vi "Get Attribute I32.vi"(8 "error in":errorcluster, 10 "Attribute":string, 11 "Config from Excel Table in":refnum<class "Config from Excel Table.lvclass">) -> (0 "error out":errorcluster, 2 "Value":i32, 3 "Config from Excel Table out":refnum<class "Config from Excel Table.lvclass">)   [LabVIEW 2025, in "Config from Excel Table.lvclass"]
uses:
  Config from Excel Table.lvclass
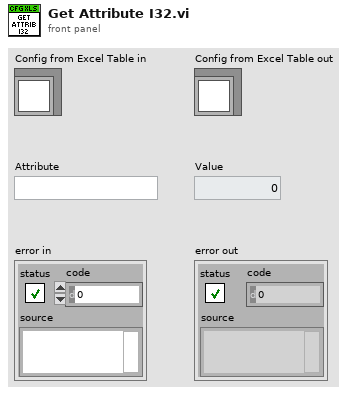
[diagram p1: front panel]
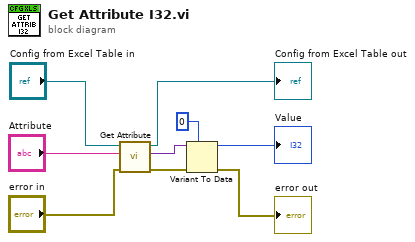
[diagram p0: block diagram]
diagram:
  n1 = call "Get Attribute.vi"("error in"="error in", "Attribute"="Attribute", "Config from EXCEL Table in"="Config from Excel Table in") -> ("error out"=w7:errorcluster, "Value"=w1:variant, "Config from EXCEL Table out"=→"Config from Excel Table out":refnum<class "Config from Excel Table.lvclass">)  [unwired: 6 in]
  n2 = Variant To Data(error in=w7, type=0, Variant=w1) -> (data=→"Value":i32, error out=→"error out":errorcluster)
